vi "Save Parameter File.vi"(8 "error in":errorcluster, 9 "mode (Create)":i32(ring)=2 items=["CreateNew"=1, "Create"=2, "Open"=3, "OpenOrCreate"=4, "Truncate"=5, "Append"=6], 10 "XML path":path, 11 "parameter file in":refnum<k24>) -> (0 "error out":errorcluster, 2 "SerializeXML":bool, 3 "parameter file out":refnum<k24>)   [LabVIEW 2020, in "AIM_Parameter_ni.lvlib"]
uses:
  AIM_Parameter_ni.lvlib
  C:/Users/Administrator/Desktop/GIT/Ballard-Arinc-429-XML-Generator/Source/Assemblies/Aim_Parameter_ni/bin/Debug/AIM_429_Parameter_ni.dll
  Assemblies/Aim_Parameter_ni/bin/Debug/AIM_429_Parameter_ni.dll
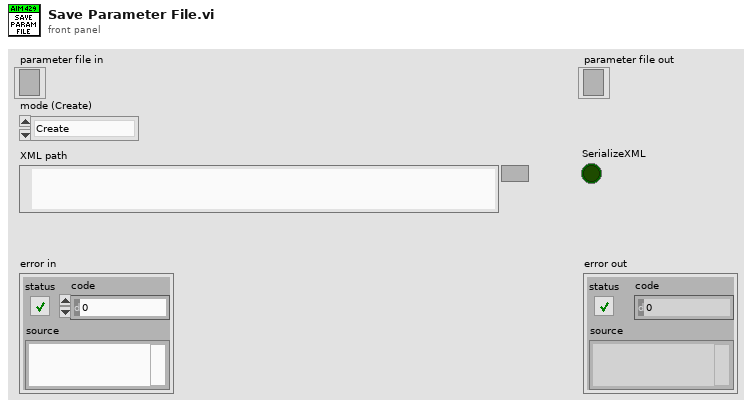
[diagram p1: front panel]
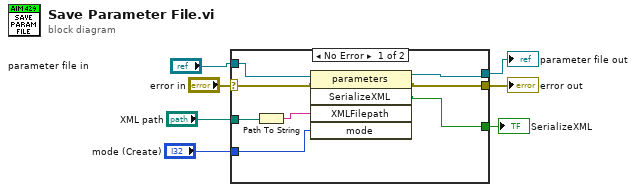
[diagram p0: block diagram]
diagram:
  n1 = case shown="No Error" "error in" {
    selector: "error in" -> [w13 w16]
    tunnel: [w10 w17] -> w7
    tunnel: [w11 w16] -> w6
    tunnel: "parameter file in" -> [w14 w17]
    tunnel: "XML path" -> [w15 _]
    tunnel: [w12 _] -> w2
    tunnel: "mode (Create)" -> [w8 _]
    frame No Error {
      n2 = Path To String(path=w15) -> (string=w9:string)
      n3 = invoke class="parameters" method="SerializeXML"(reference=w14, error in=w13, "XMLFilepath"=w9, "mode"=w8) -> (reference out=w10:refnum<k24>, error out=w11:errorcluster, "SerializeXML"=w12:bool)  [unwired: 1 in, 2 out]
    }
    frame Error {
    }
  }
  "parameter file out" <- w7
  "error out" <- w6
  "SerializeXML" <- w2
